vi "Merge.vi"(8 "error in (no error)":errorcluster, 9 "Destination":string[](array[string]), 10 "Source Tree":refnum<class "Value Tree.lvclass">, 11 "Value Tree in":refnum<class "Value Tree.lvclass">) -> (0 "error out":errorcluster, 3 "Value Tree out":refnum<class "Value Tree.lvclass">)   [LabVIEW 2020, in "HTTP Server.lvlib" / "Value Tree.lvclass"]
uses:
  Value Tree.lvclass
  Value Tree.lvclass/Value Tree.ctl
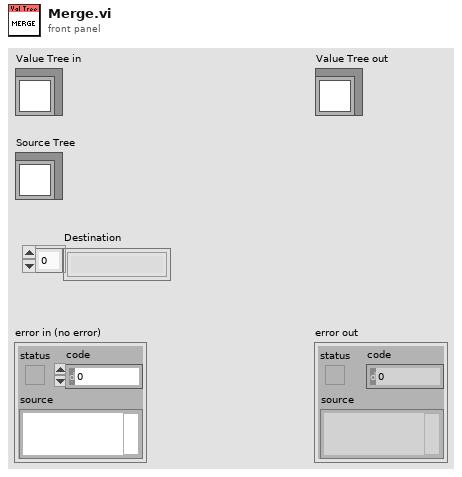
[diagram p1: front panel]
types:
  T1 = typedef "HTTP Server.lvlib/Value Tree.lvclass/Local Type.ctl" = enum16{"Scalar", "Object", "Array"}
  T2 = typedef "HTTP Server.lvlib/Value Tree.lvclass/Local Info.ctl" = cluster{"Type":T1, "Value":string, "Children":string[], "Size":i32}
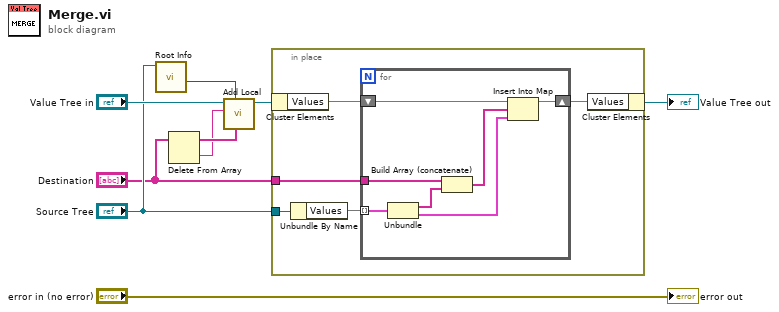
[diagram p0: block diagram]
diagram:
  n1 = call "Root Info.vi"("Value Tree in"="Source Tree") -> ("Type"=w4:T1)  [unwired: 6 in, 4 out]
  n2 = Delete From Array(array="Destination") -> (deleted portion=w1:string, array with subset deleted=w2:string[])  [unwired: 2 in]
  n3 = call "Add Local.vi"("Parent"=w2, "Type"=w4, "Name"=w1, "TemplateLocals in"="Value Tree in") -> ("TemplateLocals out"=w6:refnum<class "Value Tree.lvclass">)  [unwired: 5 in, 2 out]
  n4 = in-place {
    in-place-border: "Source Tree" -> [w12]
    in-place-border: "Destination" -> [w10]
    n5 = in-place-cluster #1(w6) -> ("Values"=w14:map{string[], T2})
    n6 = Unbundle By Name(w12) -> ("Values"=w11:map{string[], T2})
    n7 = for {
      shift-right: [w15] -> w13
      shift-left: w14 -> [w18]
      tunnel: w11 -> [w21] mode=indexing
      tunnel: w10 -> [w20]
      n8 = Unbundle(w21) -> ("Hierarchy"=w19:string[], "Info"=w16:T2)
      n9 = Build Array (concatenate)(w20, w19) -> (w17:string[])
      n10 = Insert Into Map(map in=w18, key=w17, value=w16) -> (map out=w15:map{string[], T2})  [unwired: 2 out]
    }
    n11 = in-place-cluster #1("Values"=w13) -> (→"Value Tree out":refnum<class "Value Tree.lvclass">)
  }
  "error out" <- "error in (no error)"
